vi "TractionModule Selection.vi"(8 "error in (no error)":errorcluster, 11 "Data Cluster":T1) -> (0 "error out":errorcluster)   [LabVIEW 2025]
uses:
  controls/LAB-IQ UI Data.ctl
  Traction Loop/Traction Receipe Enum.ctl
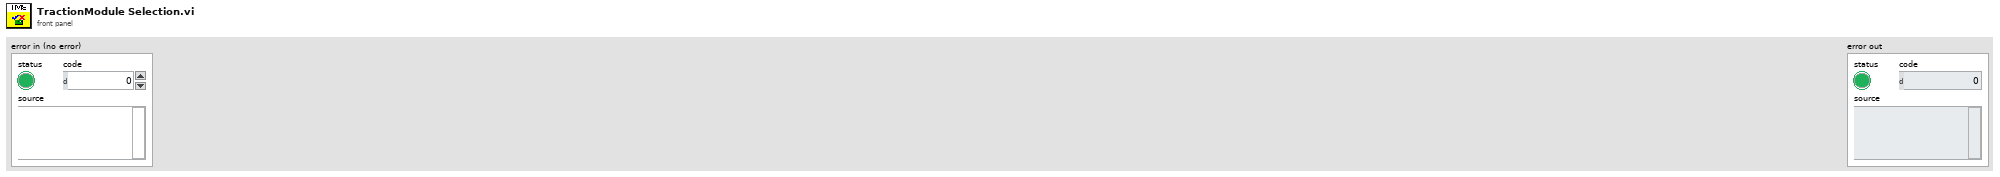
[diagram p1: front panel]
types:
  T1 = typedef "LAB-IQ UI Data.ctl" = cluster{"Main Home Screen":cluster{"GUI":refnum<vi>, "Platform Settings":refnum<vi>, "Configure":refnum<vi>, "Home":refnum<vi>, "EXIT":refnum<vi>, "service 2":refnum<vi>, "MainPage":refnum<vi>, "Analysis":refnum<vi>}, "Platform Settings":cluster{"mm/s  Surge":refnum<vi>, "Update Surge Speed":refnum<vi>, "Drive Error":refnum<vi>, "Disable Axis Jog Soft Limits":refnum<vi>, "mm/s  Sway":refnum<vi>, "Sway and Surge COM Status":refnum<vi>, "Heave COM Status":refnum<vi>, "Enable Platform":refnum<vi>, "Surge Forward Main":refnum<vi>, "Sway Right Main":refnum<vi>, "Sway Left Main":refnum<vi>, "Heave Down Main":refnum<vi>, "Heave Up main":refnum<vi>, "Update Sway Speed":refnum<vi>, "Update Heave Speed":refnum<vi>, "mm/s Heave":refnum<vi>, "mm/sec":refnum<vi>, "mm":refnum<vi>, "Surge Backward Main":refnum<vi>}, "Analysis Screen":cluster{"Analysis Home":refnum<vi>, "Surface Analysis":refnum<vi>, "Imaging":refnum<vi>, "Image Analysis":refnum<vi>, "Post Analysis":refnum<vi>}, "Config Screen":cluster{"Select Load Head":refnum<vi>, "Notes :":refnum<vi>, "FILE":refnum<vi>, "Sample ID :":refnum<vi>, "Operator ID :":refnum<vi>, "Operator Name :":refnum<vi>, "Auto":refnum<vi>}, "Motion Module":cluster{"zNL":refnum<vi>, "NL disp":refnum<vi>, "Rotary Tab":refnum<vi>, "Motion Direction:  3":refnum<vi>, "E.Velocity 2":refnum<vi>, "e.v/ssr 2":refnum<vi>, "Enter Fixed E.Velocity 2":refnum<vi>, "Enter Final SRR 2":refnum<vi>, "Enter initial SRR 2":refnum<vi>, "Enter Fixed SRR 2":refnum<vi>, "Enter the Final E.Velocity (m/s) 2":refnum<vi>, "Enter initial E.Velocity (m/s) 2":refnum<vi>, "Final Speed (RPM) 3":refnum<vi>, "Initial Speed (RPM) 2":refnum<vi>, "Enter the Final Velocity (m/s) 3":refnum<vi>, "Enter initial Velocity (m/s)  3":refnum<vi>, "Ramp Up 2":refnum<vi>, "TEST SELECTION":refnum<vi>, "SPEED SELECTION : ":refnum<vi>, "Angular Oscillation Set":refnum<vi>, "Traction":refnum<vi>, "Step Speed":refnum<vi>, "StepTable For Load-Speed":refnum<vi>, "StepTable For Speed":refnum<vi>, "Surge Forward MM":refnum<vi>, "Surge Backward MM":refnum<vi>, "M3 Image":refnum<vi>, "String 39":refnum<vi>, "Sway Left MM":refnum<vi>, "Sway Right MM":refnum<vi>, "Disable Axis Jog Soft Limits":refnum<vi>, "mm":refnum<vi>, "Heave Down MM":refnum<vi>, "Heave Up MM":refnum<vi>, "Wear Track Diameter (mm)":refnum<vi>, "Set WTD":refnum<vi>, "HomeScratch":refnum<vi>, "HomeRot":refnum<vi>, "PlaceModule":refnum<vi>, "Enter the Angle (Deg)":refnum<vi>, "Enter the Frequency (Hz)":refnum<vi>, "Motion Mode:":refnum<vi>, "LR Sway":refnum<vi>, "Rot Hor":refnum<vi>, "Scratch":refnum<vi>, "LR Cam":refnum<vi>, "MMBack":refnum<vi>, "MMNext":refnum<vi>, "Rot Ver":refnum<vi>, "Rotary Module Selection":refnum<vi>, "calculate rotary":refnum<vi>, "SPEED SELECTION : rotary":refnum<vi>, "Import 2":refnum<vi>, "Save 2":refnum<vi>, "File Path :  2":refnum<vi>, "String 45":refnum<vi>, "StepTable For Speed 3":refnum<vi>, "Enter the Speed(mm/sec)":refnum<vi>, "Enter the Speed(RPM)":refnum<vi>, "Enter Scratch Speed (mm/s):":refnum<vi>, "SwaySpeed Set":refnum<vi>, "Scartch Offset":refnum<vi>, "Motion type:":refnum<vi>, "HomeScratch 2":refnum<vi>, "Enter Scratch length (mm):":refnum<vi>, "Wear Track Diameter":refnum<vi>, "Rotary Speed Exced":refnum<vi>, "Scratch Mode":refnum<vi>, "No of Scratch":refnum<vi>}, "Environmental control":cluster{"Humidity  Status  3":refnum<vi>, "Low Temp  Status  2":refnum<vi>, "TK4 status 2":refnum<vi>, "Stage Temperature":refnum<vi>, "Sample Temperature":refnum<vi>, "Humidity (Amb)":refnum<vi>, "Clear List":refnum<vi>, "Add to list":refnum<vi>, "Wear":refnum<vi>, "Vibration":refnum<vi>, "Humidity (Chamber)":refnum<vi>, "Temperature (Chamber)":refnum<vi>, "ECR ":refnum<vi>, "Temperature (Amb)":refnum<vi>, "Microphone":refnum<vi>, "Acoustic Emission 3":refnum<vi>, "SNext":refnum<vi>, "APBack":refnum<vi>, "Enter the Temperature (°C):":refnum<vi>, "Enter the Stage \nTemperature (°C):":refnum<vi>, "Enter the Humidity (%Rh):":refnum<vi>, "Low Temp":refnum<vi>, "High Temp":refnum<vi>, "Humidity":refnum<vi>, "Sensors Picked":refnum<vi>}, "About Screen":cluster{"Password":refnum<vi>, "Home Service":refnum<vi>, "Advanced Setting":refnum<vi>, "About Tab":refnum<vi>, "ECR Port:":refnum<vi>, "Ramp Port:":refnum<vi>, "Installation/Replacement completed":refnum<vi>, "Loahead":refnum<vi>, "Heave and Surge COM Port:":refnum<vi>, "Sway COM Port:":refnum<vi>, "Temp Modbus:":refnum<vi>, "Humidity Port:":refnum<vi>, "Edit Gain Constants":refnum<vi>, "Save Gain Constants":refnum<vi>}, "Main Screen":cluster{"Main Screen Tab":refnum<vi>, "Angle and Frequency":refnum<vi>, "Stroke (mm)":refnum<vi>, "Angle (Deg)":refnum<vi>, "Main Speed Tab":refnum<vi>, "MTM MOTOR DISPLAY":refnum<vi>, "Disc Speed (m/sec)":refnum<vi>, "Ball Speed (m/sec)":refnum<vi>, "Disc Speed (RPM)":refnum<vi>, "Ball Speed (RPM)":refnum<vi>, "SPEED TAB":refnum<vi>, "Speed (m/sec)":refnum<vi>, "Set Speed (m/sec)":refnum<vi>, "Speed (RPM)":refnum<vi>, "Set Speed":refnum<vi>, "Time Tab":refnum<vi>, "Time ( HH:MM:SS ) 2":refnum<vi>, "Test Duration":refnum<vi>, "Test Duration 4":refnum<vi>, "TEST CYCLE":refnum<vi>, "TOTAL CYCLES":refnum<vi>, "Set Load (N)":refnum<vi>, "Temp Tabs":refnum<vi>, "Heater":refnum<vi>, "TK4 status":refnum<vi>, "ChamberTemp":refnum<vi>, "SetTmp":refnum<vi>, "Controller  Status":refnum<vi>, "ChamberTemp 2":refnum<vi>, "SetTmp 2":refnum<vi>, "Controller  Status 2":refnum<vi>, "ChamberTemp 3":refnum<vi>, "SetTmp 3":refnum<vi>, "Cooling":refnum<vi>, "Load Communication":refnum<vi>, "Ambient \nTemperature":refnum<vi>, "HumCOMStatus":refnum<vi>, "Ambient\n Humidity":refnum<vi>, "Freq (Hz)":refnum<vi>, "Load En":refnum<vi>, "NLt":refnum<vi>, "zNL 2":refnum<vi>, "Humidity On":refnum<vi>, "humidity disp":refnum<vi>, "Set Humidity":refnum<vi>, "NL disp 2":refnum<vi>, "Humidity On 2":refnum<vi>, "humidity disp 2":refnum<vi>, "Set Humidity 2":refnum<vi>, "NL disp 3":refnum<vi>, "AppLoadSeq scratch":refnum<vi>, "Stop Scratch":refnum<vi>, "ClrLog":refnum<vi>, "Trip Log":refnum<vi>, "STOP":refnum<vi>, "Start Test":refnum<vi>, "Test status":refnum<vi>, "AR Led":refnum<vi>, "Data":refnum<vi>, "Health":refnum<vi>, "Sway COM Status":refnum<vi>, "Heave COM Status":refnum<vi>, "Grp Tab":refnum<vi>, "Sub Graph":refnum<vi>, "SD (mm)":refnum<vi>, "Siliding distance Reset Graph":refnum<vi>, "SDGp":refnum<vi>, "Humidity Reset Graph":refnum<vi>, "HumrGp":refnum<vi>, "Acoustic Emission (mV)":refnum<vi>, "Aqucostic Reset Graph":refnum<vi>, "gACQUOS":refnum<vi>, "ECR RESET":refnum<vi>, "ECR":refnum<vi>, "Temperature Reset":refnum<vi>, "Acoustic Emission (mV) 2":refnum<vi>, "Aqucostic Reset Graph 2":refnum<vi>, "gACQUOS 2":refnum<vi>, "ECR RESET 2":refnum<vi>, "ECR 2":refnum<vi>, "Temperature Reset 2":refnum<vi>, "Temperature (deg c)":refnum<vi>, "Speed Reset Graph":refnum<vi>, "Speed Tab":refnum<vi>, "MTM DISC  SPEED":refnum<vi>, "MTM BALL SPEED":refnum<vi>, "speed mm/sec":refnum<vi>, "Hymidity":refnum<vi>, "Humidity Disable trip":refnum<vi>, "CoF Trip  2":refnum<vi>, "Depth Trip":refnum<vi>, "Weart Deapth":refnum<vi>, "Depth Reset Graph":refnum<vi>, "Weart":refnum<vi>, "Depthz":refnum<vi>, "Depth (µm)":refnum<vi>, "WearGp":refnum<vi>, "NL Trip 2":refnum<vi>, "Load pid":refnum<vi>, "Load Disable Trip":refnum<vi>, "Load Reset Graph":refnum<vi>, "NL Display 4":refnum<vi>, "Main Chart 3":refnum<vi>, "BACK":refnum<vi>, "Depth Trip 2":refnum<vi>, "COF TRIP ":refnum<vi>, "Friction Force (N)":refnum<vi>, "FF Reset Graph":refnum<vi>, "FF Disable Trip":refnum<vi>, "FF TRIP":refnum<vi>, "COF Disable Trip":refnum<vi>, "COF Reset Graph":refnum<vi>, "Start Test Temp":refnum<vi>, "zFF":refnum<vi>, "Friction Force (N) Graph":refnum<vi>, "Coefficient of Friction":refnum<vi>, "Scratch Start Test":refnum<vi>, "FF Tab":refnum<vi>, "Cyclic Friction Force (N)":refnum<vi>, "CZ FF":refnum<vi>, "Cyclic Friction Force (N) Graph":refnum<vi>, "Cyclic Coefficient of Friction":refnum<vi>, "Cyclic FF TRIP":refnum<vi>, "Cyclic FF Disable Trip":refnum<vi>, "cyclic COF Disable Trip":refnum<vi>, "cyclic COF TRIP":refnum<vi>, "cyclic COF Reset Graph":refnum<vi>, "Cyclic FF Reset Graph":refnum<vi>, "Test Trip":refnum<vi>, "Multi Scratch Pass":refnum<vi>, "Scratch Start Recording":refnum<vi>}, "Loading":cluster{"Indentation":refnum<vi>, "Reference Sample":refnum<vi>, "Load Cell Communication Slide":refnum<vi>, "com 3":refnum<vi>, "com":refnum<vi>, "DecaForce COM Status":refnum<vi>, "Update":refnum<vi>, "Clear 3":refnum<vi>, "seq":refnum<vi>, "Stribeck table":refnum<vi>, "Stribeck Table  For loading":refnum<vi>, "Loading Mode":refnum<vi>, "Enter the Final Load (N)":refnum<vi>, "Enter the CoF Trip":refnum<vi>, "Enter the Friction Force Trip":refnum<vi>, "Enter the Normal load Trip":refnum<vi>, "Enter the Load  (N)":refnum<vi>, "KiloForce":refnum<vi>, "DecaForce ":refnum<vi>, "MicroForce":refnum<vi>, "LHBack":refnum<vi>, "LHNext":refnum<vi>, "Enter the Loading Rate (N/min)":refnum<vi>, "Message":refnum<vi>, "Warning 2":refnum<vi>, "SSP 0.75":refnum<vi>, "SSP 0.5":refnum<vi>, "SSP 0.3":refnum<vi>, "Warning":refnum<vi>, "gui GIF":refnum<vi>, "Communication is established":refnum<vi>, "AppLoad 4":refnum<vi>, "Multipoint":refnum<vi>, "Load Selection":refnum<vi>}, "PID":cluster{"Ramp MulFac":refnum<vi>, "pulses LoadDiffRamp(2..10)":refnum<vi>, "PulseControlRamp(diff<=3N)":refnum<vi>, "SetLoadDeadband(%) Load(0-10N)":refnum<vi>, "PID gains out delay (microForce)":refnum<vi>, "Ramp":refnum<vi>, "Gain 2":refnum<vi>, "pulses LoadDiff(2..10)":refnum<vi>, "pulses LoadDiff(11..50)":refnum<vi>, "PulseControl(diff<=3N)":refnum<vi>, "SetLoadDeadband(%)  2":refnum<vi>, "Dummy Run":refnum<vi>, "Vertical load (N)":refnum<vi>, "AutoTune":refnum<vi>, "Offset 3 ":refnum<vi>, "apply load":refnum<vi>, "Offset  3":refnum<vi>, "apply load 2":refnum<vi>, "Enter ByPass Load":refnum<vi>, "reinit 3":refnum<vi>, "output range delay":refnum<vi>, "PID gains out delay":refnum<vi>, "Bypass Load":refnum<vi>, "pulsesSent":refnum<vi>, "pulses ":refnum<vi>, "actpid":refnum<vi>, "gFF Rot":refnum<vi>, "pulses LoadDiff(21..1000)":refnum<vi>, "Delay":refnum<vi>, "deadband":refnum<vi>}, "Config Parameters":cluster{"Tab Control 3":refnum<vi>, "Tab Control 19":refnum<vi>, "SAMPLES":refnum<vi>, "Re-initilaize":refnum<vi>, "Filter ON/OFF":refnum<vi>, "TracHomeSurgeOffsetCounts 10MM":refnum<vi>, "TracHomeSwayOffsetCounts 10MM":refnum<vi>, "Acoustic Emission:":refnum<vi>, "Apply Filter (FF)":refnum<vi>, "Filter% 2":refnum<vi>, "Apply Filter (Load)":refnum<vi>, "Filter% ":refnum<vi>, "Sway distance (mm)":refnum<vi>, "Surge distance (mm)":refnum<vi>, "DataSavingLoopDelay(ms)":refnum<vi>, "SAVE 2":refnum<vi>, "Enter Distance":refnum<vi>, "Sway Counts:":refnum<vi>, "Distance (mm): 3":refnum<vi>, "Surge Counts:":refnum<vi>, "Distance (mm): 2":refnum<vi>, "Distance (mm):":refnum<vi>, "Heave Counts:":refnum<vi>, "LRMHomeSurgeOffsetCounts":refnum<vi>, "LRMHomeSwayOffsetCounts":refnum<vi>, "TracHomeSurgeOffsetCounts 20MM":refnum<vi>, "TracHomeSwayOffsetCounts 20MM":refnum<vi>, "RotHomeSwayOffsetCounts":refnum<vi>, "RotHomeSurgeOffsetCounts":refnum<vi>, "Heave distance":refnum<vi>, "Zmm":refnum<vi>, "Heave Pulses/mm":refnum<vi>, "Surge Pulses/mm":refnum<vi>, "Sway Pulses/mm":refnum<vi>, "Heave Pitch":refnum<vi>, "Surge Pitch":refnum<vi>, "Sway Pitch":refnum<vi>, "Heave PPR":refnum<vi>, "Surge PPR":refnum<vi>, "Sway PPR":refnum<vi>, "Tab Control 5":refnum<vi>, "Tab Control 14":refnum<vi>, "Tab Control 26":refnum<vi>, "AE":refnum<vi>, "Heave Loop Delay":refnum<vi>, "Heave PID Speed":refnum<vi>, "Surge Jog Speed":refnum<vi>, "Heave Jog Speed":refnum<vi>, "Sway Loop Delay":refnum<vi>, "Sway PID Speed":refnum<vi>, "Sway Jog Speed":refnum<vi>, "DEPTH TRIP VALUE":refnum<vi>, "LOAD TRIP VALUE":refnum<vi>, "DEPTH TRIP   ENABLE":refnum<vi>, "LOAD TRIP  ENABLE":refnum<vi>, "CYCLIC FF TRIP VALUE":refnum<vi>, "FF TRIP VALUE":refnum<vi>, "CYCLIC CoF TRIP VALUE":refnum<vi>, "COF TRIP VALUE":refnum<vi>, "CYCLIC COF TRIP  ENABLE":refnum<vi>, "CYCLIC FF TRIP  ENABLE":refnum<vi>, "FF TRIP  ENABLE":refnum<vi>, "COF TRIP  ENABLE":refnum<vi>, "JOG TRIP LOAD VALUE (N)":refnum<vi>, "Rotary Vertical":refnum<vi>, "Traction":refnum<vi>, "Scratch":refnum<vi>, "LRM CAM":refnum<vi>, "Sway LRM":refnum<vi>, "Rotary Horizontal":refnum<vi>}, "Loading Com Port":cluster{"ClearAll":refnum<vi>, "Mz(Nm)":refnum<vi>, "My(Nm)":refnum<vi>, "Mx(Nm)":refnum<vi>, "Save Dwell":refnum<vi>, "Acq Delay (ms)":refnum<vi>, "Burst Delay (ms)":refnum<vi>, "model":refnum<vi>, "SN":refnum<vi>, "FFx(N)":refnum<vi>, "Sensor IP":refnum<vi>, "Port":refnum<vi>, "FFy(N)":refnum<vi>, "Load(N)":refnum<vi>, "delete Handle":refnum<vi>, "Create Handle":refnum<vi>, "ft_data":refnum<vi>, "ft_range":refnum<vi>, "ft_data 2":refnum<vi>, "stop 6":refnum<vi>, "running_flag":refnum<vi>, "ft_udp_handle":refnum<vi>, "get-data-return":refnum<vi>, "get-range-return":refnum<vi>, "zero-return":refnum<vi>, "filter-return":refnum<vi>, "initial-return":refnum<vi>, "deleteHandle-result":refnum<vi>, "Load Cell Temp":refnum<vi>, "Load Cell":refnum<vi>, "ZeroAll":refnum<vi>, "FORCE (N)":refnum<vi>, "TORQUE (N-m)":refnum<vi>}, "Heave AND Surge":cluster{"SURGE POSE":refnum<vi>, "error out Read":refnum<vi>, "HEAVE POSE":refnum<vi>, "State":refnum<vi>, "Homed":refnum<vi>, "Sequence ID":refnum<vi>, "error out Write":refnum<vi>, "faultCode":refnum<vi>, "Ack ID":refnum<vi>, "SPEED":refnum<vi>, "Distance":refnum<vi>, "Mode Command":refnum<vi>, "Heave and Surge Read":refnum<vi>, "Read Heave Temp":refnum<vi>, "Spare 15":refnum<vi>, "Spare 14":refnum<vi>, "Spare 13":refnum<vi>, "Spare 12":refnum<vi>, "Spare 11":refnum<vi>, "Spare 10":refnum<vi>, "Spare 9":refnum<vi>, "Spare 8":refnum<vi>, "Spare 7":refnum<vi>, "Spare 6":refnum<vi>, "Spare 5":refnum<vi>, "Spare 4":refnum<vi>, "Spare 2":refnum<vi>, "Spare 1":refnum<vi>, "Node Id":refnum<vi>, "Spare 3":refnum<vi>, "SPARE 4":refnum<vi>, "SPARE 3":refnum<vi>, "SPARE 2":refnum<vi>, "SPARE 1":refnum<vi>, "fwMajor":refnum<vi>, "fwMinor":refnum<vi>, "Manual Write":refnum<vi>, "Heave and Surge Write":refnum<vi>, "SPARE 5":refnum<vi>, "Reserved ":refnum<vi>, "SPARE 8":refnum<vi>, "SPARE 6":refnum<vi>, "SPARE 7":refnum<vi>, "SPARE 17":refnum<vi>, "SPARE 16":refnum<vi>, "SPARE 15":refnum<vi>, "SPARE 14":refnum<vi>, "SPARE 13":refnum<vi>, "SPARE 12":refnum<vi>, "SPARE 11":refnum<vi>, "SPARE 10":refnum<vi>, "SPARE 9":refnum<vi>, "System UPTIME":refnum<vi>, "Missed Packets":refnum<vi>, "faultCode Surge Right":refnum<vi>, "faultCode Surge Left":refnum<vi>, "faultCode Heave":refnum<vi>, "UPLINK HEAVE":refnum<vi>, "DOWNLINK HEAVE":refnum<vi>}, "New PID LOGIC":cluster{"Fine Tune Zone":refnum<vi>, "PID SDelay":refnum<vi>, "Max_pos_limit":refnum<vi>, "Min_pos_limit":refnum<vi>, "i_limit":refnum<vi>, "pct_scale":refnum<vi>, "Deadband":refnum<vi>, "Kd":refnum<vi>, "Ki":refnum<vi>, "Kp":refnum<vi>, "Current Position":refnum<vi>, "Set Load":refnum<vi>, "Current Load":refnum<vi>, "Pulse delta":refnum<vi>, "Init Step":refnum<vi>, "Max Step Linit":refnum<vi>, "min_deadband_floor":refnum<vi>, "dynamic_spindle_noise_scalar":refnum<vi>, "min_finetune_floor":refnum<vi>, "filter_alpha":refnum<vi>, "PID":refnum<vi>}, "SWAY ":cluster{"fwMajor":refnum<vi>, "Homed":refnum<vi>, "Rotary POSE":refnum<vi>, "State":refnum<vi>, "SWAY POSE":refnum<vi>, "Ack ID":refnum<vi>, "faultCode":refnum<vi>, "Node Id":refnum<vi>, "fwMinor":refnum<vi>, "Spare 6":refnum<vi>, "Spare 5":refnum<vi>, "Spare 4":refnum<vi>, "Spare 3":refnum<vi>, "Spare 2":refnum<vi>, "Spare 1":refnum<vi>, "Spare 7":refnum<vi>, "SPARE  5":refnum<vi>, "error out Write  SWAY ":refnum<vi>, "error out Read SWAY ":refnum<vi>, "Manual Write SWAY ":refnum<vi>, "SWAY WRITE":refnum<vi>, "SPARE  4":refnum<vi>, "SPARE  3":refnum<vi>, "SPARE 2":refnum<vi>, "SPARE 1":refnum<vi>, "Spare 15":refnum<vi>, "Spare 14":refnum<vi>, "Spare 13":refnum<vi>, "Spare 12":refnum<vi>, "Spare 11":refnum<vi>, "Spare 9":refnum<vi>, "Spare 8":refnum<vi>, "SPEED":refnum<vi>, "Distance":refnum<vi>, "Mode Command":refnum<vi>, "Sequence ID":refnum<vi>, "SWAY READ":refnum<vi>, "Spare 10":refnum<vi>, "Read SWAY Temp":refnum<vi>, "faultCode Sway ":refnum<vi>, "Missed Packets":refnum<vi>, "System UPTIME sway":refnum<vi>, "SPARE 6":refnum<vi>, "SPARE 7":refnum<vi>, "SPARE 9":refnum<vi>, "SPARE 11":refnum<vi>, "SPARE 10":refnum<vi>, "SPARE 8":refnum<vi>, "SPARE 13":refnum<vi>, "SPARE 12":refnum<vi>, "SPARE 17":refnum<vi>, "SPARE 16":refnum<vi>, "SPARE 15":refnum<vi>, "SPARE 14":refnum<vi>, "Reserved":refnum<vi>, "faultCode Rotary":refnum<vi>, "UPLINK SWAY":refnum<vi>, "DOWNLINK SWAY":refnum<vi>}, "Analysis Screen":cluster{"Analysis Home":refnum<vi>, "Refresh 2":refnum<vi>, "MEAN 4":refnum<vi>, "SD 4":refnum<vi>, "VARIANCE 4":refnum<vi>, "MEAN  3":refnum<vi>, "SD  3":refnum<vi>, "VARIANCE  3":refnum<vi>, "MEAN 2":refnum<vi>, "SD  2":refnum<vi>, "VARIANCE 2":refnum<vi>, "MEAN":refnum<vi>, "SD":refnum<vi>, "VARIANCE":refnum<vi>, "File 4 Discription":refnum<vi>, "OPEN 4":refnum<vi>, "File Name 4":refnum<vi>, "OPEN 3":refnum<vi>, "File 3 Discription":refnum<vi>, "File Name 3":refnum<vi>, "Y-AXIS":refnum<vi>, "X-AXIS":refnum<vi>, "XY Graph":refnum<vi>, "File Name 2":refnum<vi>, "File Name 1":refnum<vi>, "OPEN 2":refnum<vi>, "OPEN 1":refnum<vi>, "File 1 Discription ":refnum<vi>, "File 2 Discription":refnum<vi>, "Export":refnum<vi>, "File Format":refnum<vi>}, "Traction":cluster{"faultCode Traction 2":refnum<vi>, "faultCode Traction 1":refnum<vi>, "Missed Packets":refnum<vi>, "System UPTIME Traction":refnum<vi>, "SPARE 17":refnum<vi>, "SPARE 16":refnum<vi>, "SPARE 15":refnum<vi>, "SPARE 14":refnum<vi>, "SPARE 13":refnum<vi>, "SPARE 12":refnum<vi>, "SPARE 11":refnum<vi>, "SPARE 10":refnum<vi>, "SPARE 9":refnum<vi>, "SPARE 8":refnum<vi>, "SPARE 7":refnum<vi>, "SPARE 6":refnum<vi>, "Reserved":refnum<vi>, "SPARE  5":refnum<vi>, "Manual Write TRACTION":refnum<vi>, "TRACTION WRITE":refnum<vi>, "SPARE  4":refnum<vi>, "SPARE  3":refnum<vi>, "SPARE 2":refnum<vi>, "SPARE 1":refnum<vi>, "Spare 7":refnum<vi>, "Spare 6":refnum<vi>, "Spare 5":refnum<vi>, "Spare 4":refnum<vi>, "Spare 2":refnum<vi>, "Spare 1":refnum<vi>, "Node Id":refnum<vi>, "Read TRACTION Temp":refnum<vi>, "fwMinor":refnum<vi>, "fwMajor":refnum<vi>, "faultCode":refnum<vi>, "TRACTION POSE":refnum<vi>, "TRACTION POSE 2":refnum<vi>, "Homed":refnum<vi>, "State":refnum<vi>, "Ack ID":refnum<vi>, "SPEED":refnum<vi>, "Distance":refnum<vi>, "Mode Command":refnum<vi>, "Sequence ID":refnum<vi>, "error out Read TRACTION":refnum<vi>, "error out Write  TRACTION":refnum<vi>, "TRACTION READ":refnum<vi>, "Spare 3":refnum<vi>, "Downlink traction":refnum<vi>, "Uplink Traction":refnum<vi>}, "Traction reciepe":cluster{"SRR Sweep Range (%) Stribeck":refnum<vi>, "Traction Receipe":refnum<vi>, "Total Execution Time":refnum<vi>, "Total Steps":refnum<vi>, "Duration / Step (s)  Stribeck":refnum<vi>, "STRIBECK Fixed SRR List (%)":refnum<vi>, "Duration / Step (s) Traction":refnum<vi>, "SRR Sweep Range (%) traction":refnum<vi>, "Rolling Speed (mm/s)":refnum<vi>, "Temperature Stages (°C)":refnum<vi>, "Ball Load (N)":refnum<vi>, "Lubricant Name":refnum<vi>, "Profile File Name":refnum<vi>, "SET entrainment Velocity":refnum<vi>, "Test Array Size":refnum<vi>, "SRR INDEX [ STRIBECK]":refnum<vi>, "Stribeck Size":refnum<vi>, "SET SRR":refnum<vi>, "ELAPSED TIMER ":refnum<vi>, "BALL SET RPM":refnum<vi>, "DISC SET RPM":refnum<vi>, "SET LOAD":refnum<vi>, "TEMPERATURE READ":refnum<vi>, "SET TEMPERATURE":refnum<vi>, "Traction Size":refnum<vi>, "DISC SPEED (rpm)":refnum<vi>, "BALL SPEED (rpm)":refnum<vi>, "BALL WEAR TRACK":refnum<vi>, "DISC WEARTRACK":refnum<vi>, "SRR INDEX [ TRACTION]":refnum<vi>, "Start Index Type":refnum<vi>, "Enum - Menu":refnum<vi>, "Ball (mm/sec)":refnum<vi>, "Disc (mm/sec)":refnum<vi>}, "Traction Control":cluster{"HomeTraction":refnum<vi>, "Demo Mode Display":refnum<vi>, "Traction Message":refnum<vi>, "Traction Step Update Details":refnum<vi>, "Main Tab sequence for selection":refnum<vi>, "Ramp Tab":refnum<vi>, "e.v/ssr":refnum<vi>, "Enter Fixed E.Velocity":refnum<vi>, "Enter Final SRR":refnum<vi>, "Enter initial SRR":refnum<vi>, "Enter Fixed SRR":refnum<vi>, "Enter the Final E.Velocity (m/s)":refnum<vi>, "Enter initial E.Velocity (m/s)":refnum<vi>, "Ball WTD":refnum<vi>, "E.Velocity":refnum<vi>, "Enter the Final Velocity (m/s)":refnum<vi>, "Enter initial Velocity (m/s)":refnum<vi>, "Ramp Up   Disc":refnum<vi>, "Initial DiscSpeed (RPM)":refnum<vi>, "Final Speed (RPM) Ball":refnum<vi>, "Final Speed (RPM)":refnum<vi>, "Initial Speed (RPM) Ball":refnum<vi>, "Enter the Final Velocity (m/s) Ball":refnum<vi>, "Enter initial Velocity (m/s) Ball":refnum<vi>, "Ramp Up":refnum<vi>, "ExceedBallSpeed step":refnum<vi>, "ExceedDiscSpeed":refnum<vi>, "BallSpeed Exceed Indication":refnum<vi>, "Apply":refnum<vi>, "SPEED SELECTION : MTM":refnum<vi>, "SPEED SELECTION : MTM 2":refnum<vi>, "TEST SELECTION (MTM)":refnum<vi>, "MTM Test Selection":refnum<vi>, "File Path Tab":refnum<vi>, "File Path String":refnum<vi>, "Save":refnum<vi>, "Save  2":refnum<vi>, "Import ":refnum<vi>, "File Path :":refnum<vi>, "Step Sequence Indication Tab":refnum<vi>, "Step Sequence Indication":refnum<vi>, "Calculate Step":refnum<vi>, "StepTable":refnum<vi>, "ExceedDiscSpeed  Cinstant Speed":refnum<vi>, "ExceedBallSpeed Constant":refnum<vi>, "TEST SELECTION (MTM) 2":refnum<vi>, "SPEED SELECTION : MTM 3":refnum<vi>, "MTM Test Selection 2":refnum<vi>, "Enter the Speed (m/sec): ":refnum<vi>, "Enter the Speed (m/sec):  2":refnum<vi>, "Enter the Speed (RPM):":refnum<vi>, "Lower Spped ":refnum<vi>, "Upper":refnum<vi>, "Enter the Speed (RPM):Ball":refnum<vi>, "Disc Motion Direction: ":refnum<vi>, "Ball Motion Direction :":refnum<vi>, "Motion Mode: ":refnum<vi>, "Wear Track Diameter (mm) ":refnum<vi>, "Disc Speed Indicator":refnum<vi>, "ExceedBallSpeed":refnum<vi>}, "Acquostic":cluster{"Last Config Rejected ":refnum<vi>, "rx command count":refnum<vi>, "Current Filter Id":refnum<vi>, "Isolated Gain":refnum<vi>, "DAQ Status":refnum<vi>, "error out":refnum<vi>, "error in (no error)":refnum<vi>, "Uplink Packet":refnum<vi>, "data out":refnum<vi>, "Downlink Packet":refnum<vi>, "Signal Energy":refnum<vi>, "Amplitude db_AE":refnum<vi>, "Peak Amplitude":refnum<vi>, "AE Ring-Down Counts":refnum<vi>, "Gains":refnum<vi>, "Manual Write Acquostic":refnum<vi>}}
  T2 = enum32{"Details", "PlatformSetting", "Analysis", "HOME"}
  T3 = enum32{"Setup", "Load Head", "Motion Module", "Environment", "Begin"}
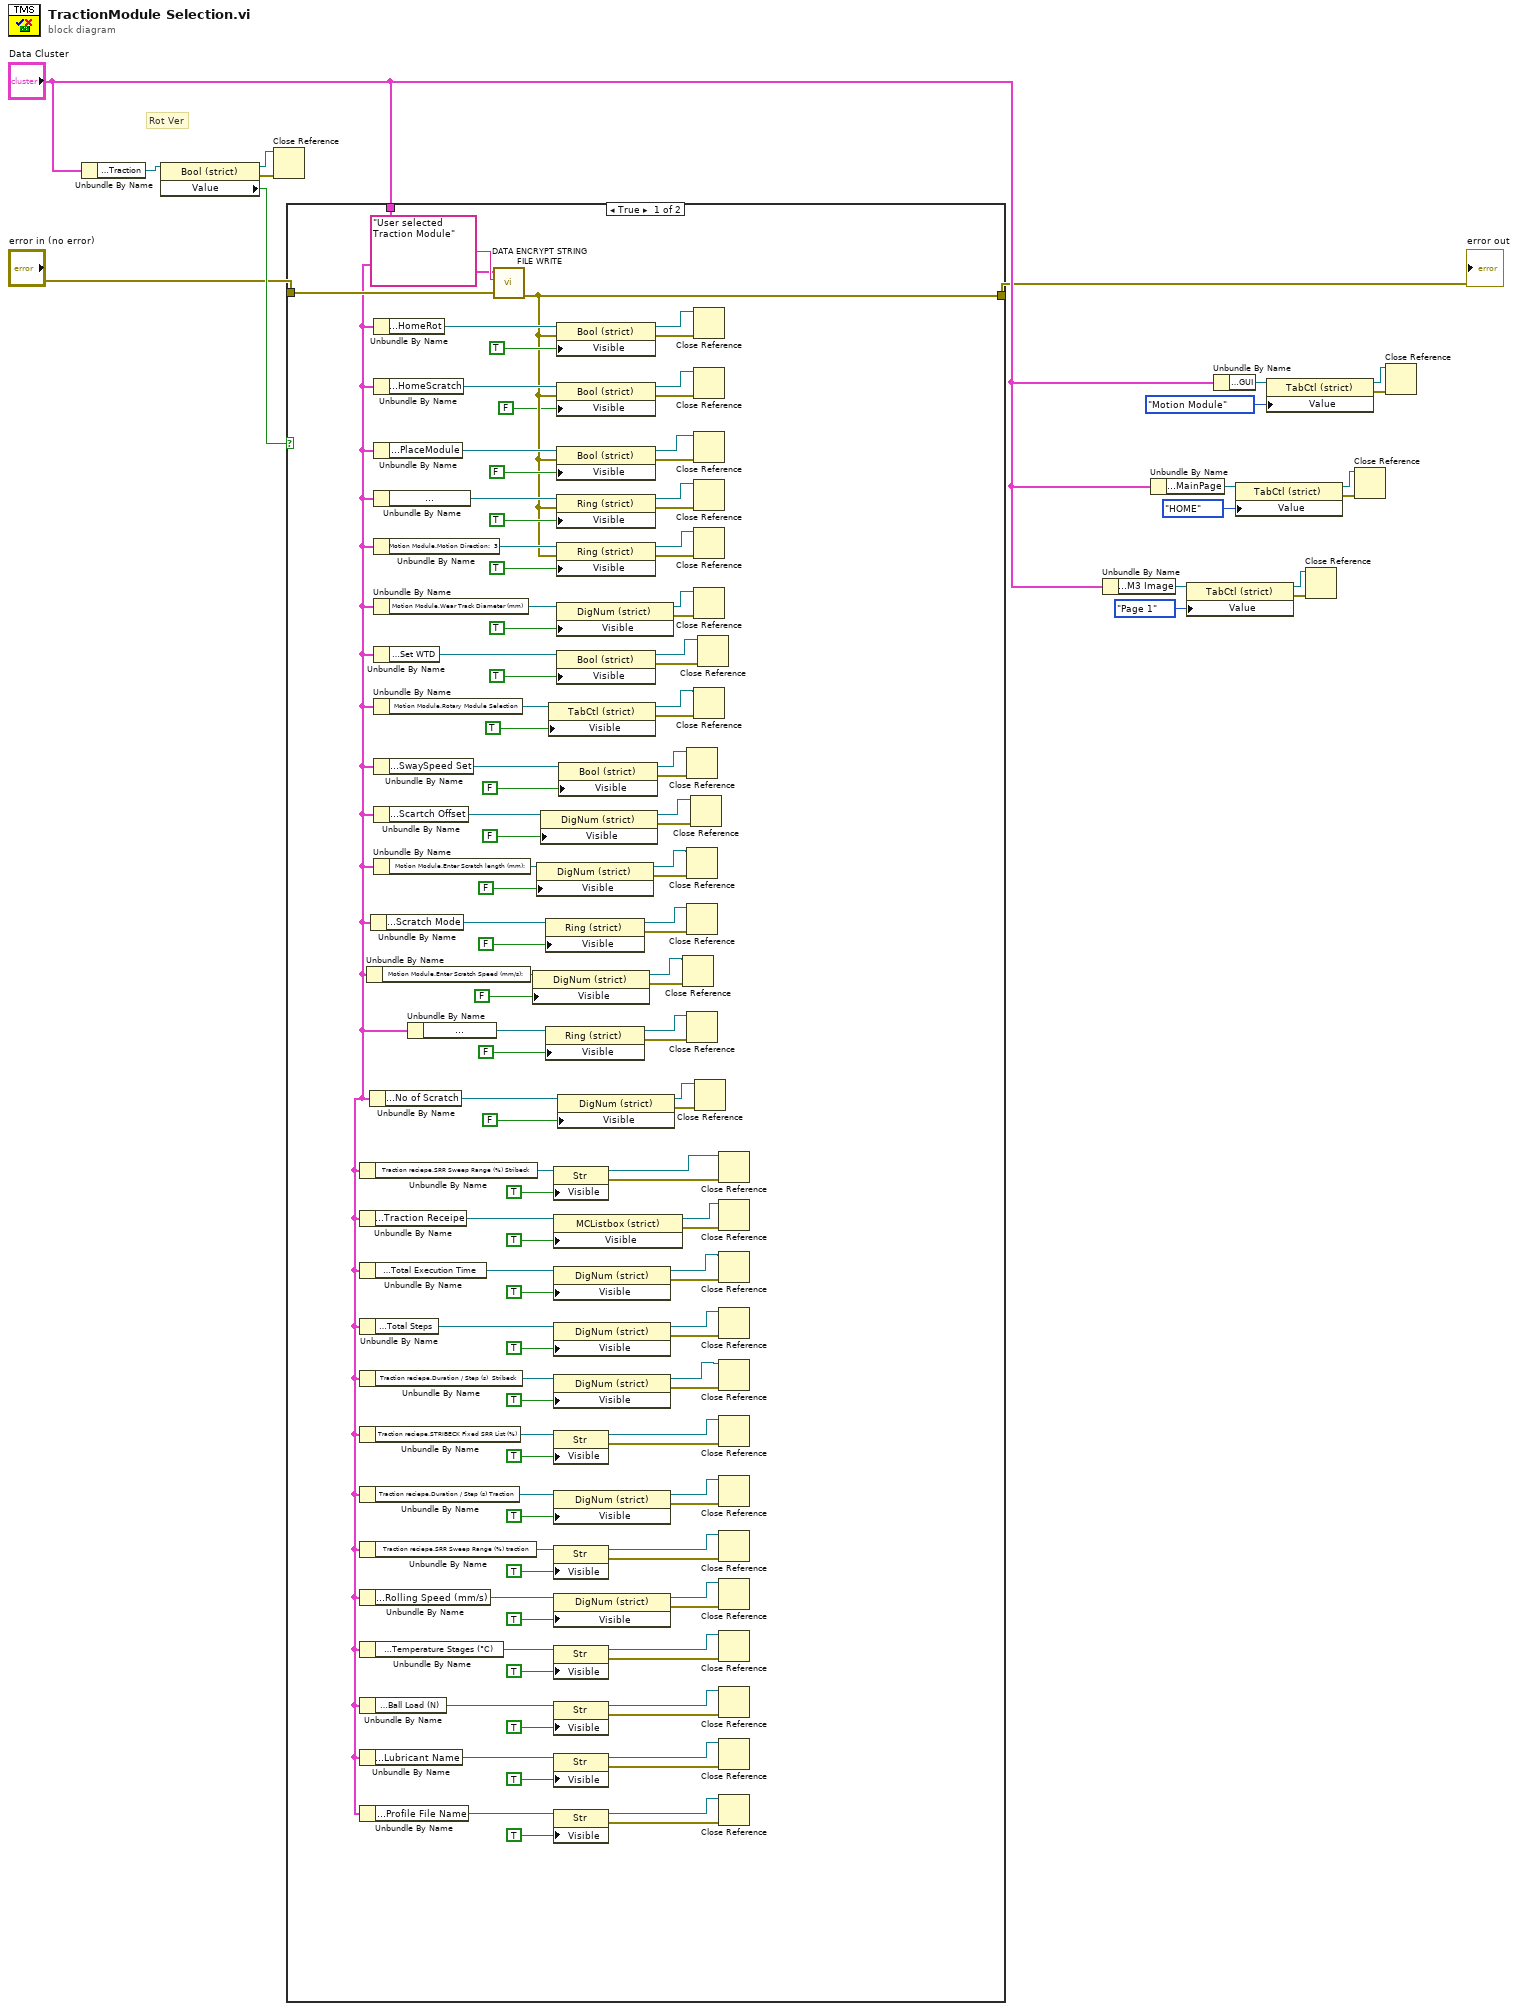
[diagram p0: block diagram]
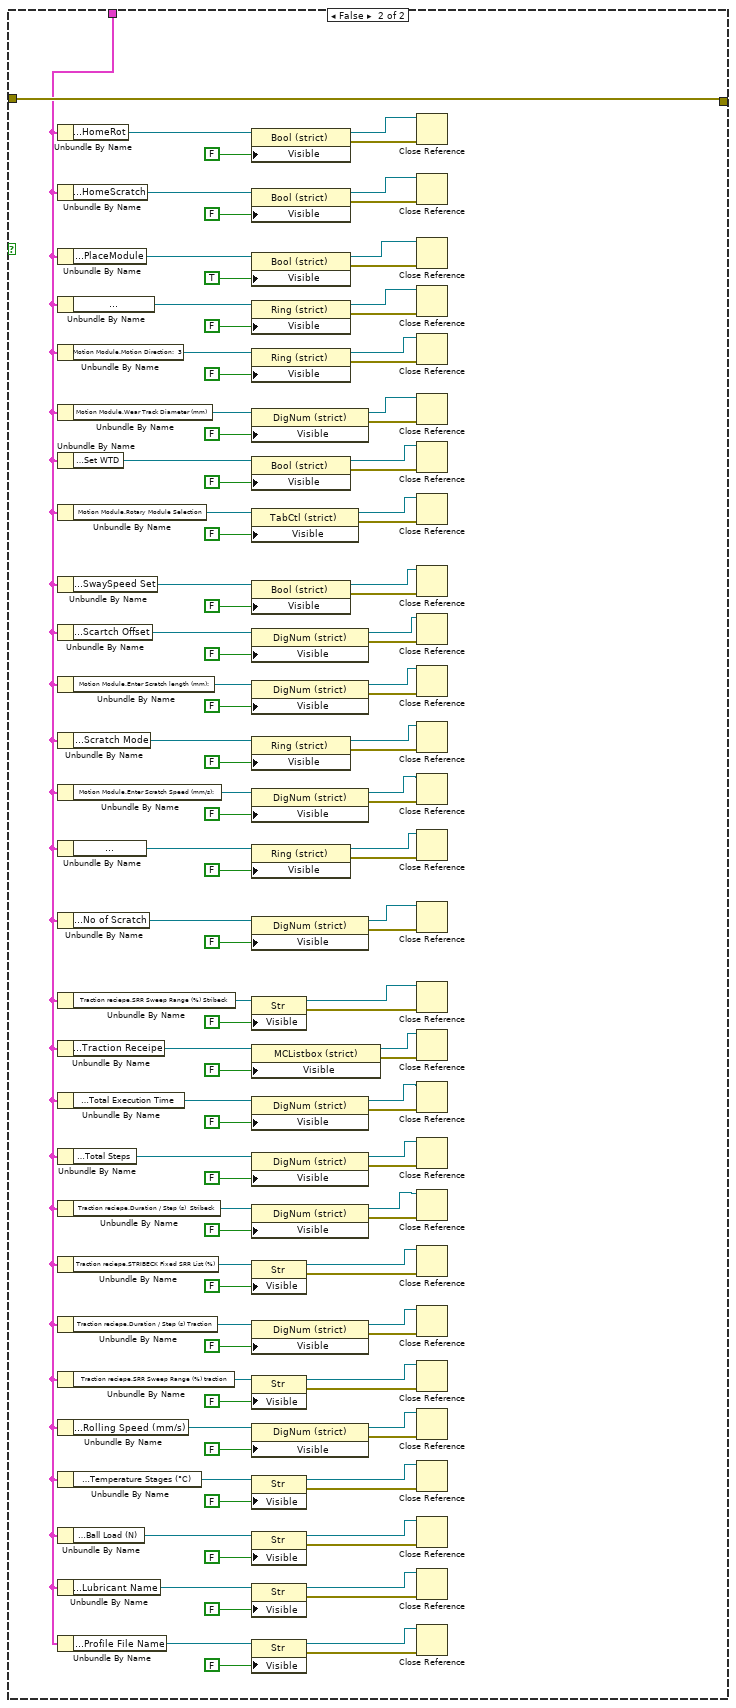
[diagram p2: hidden frame]
diagram:
  # "Rot Ver"
  n1 = Unbundle By Name("Data Cluster") -> ("Motion Module.Traction"=w18:refnum<vi>)
  n2 = property class="Bool (strict)"(reference=w18) -> (reference out=w15:refnum<vi>, error out=w16:errorcluster, "Value"=w19:bool)  [unwired: 1 in]
  n3 = Close Reference(reference=w15, error in (no error)=w16) -> ()  [unwired: 1 out]
  n4 = case shown="True" w19 {
    tunnel: "error in (no error)" -> [w134 w249]
    tunnel: [w106 w249] -> w10
    tunnel: "Data Cluster" -> [w20 w136]
    frame True {
      n5 = Unbundle By Name(w20) -> ("Traction reciepe.SRR Sweep Range (%) Stribeck"=w55:refnum<vi>)
      n6 = Unbundle By Name(w20) -> ("Traction reciepe.Traction Receipe"=w58:refnum<vi>)
      n7 = Unbundle By Name(w20) -> ("Traction reciepe.Total Execution Time"=w61:refnum<vi>)
      n8 = Unbundle By Name(w20) -> ("Traction reciepe.Total Steps"=w53:refnum<vi>)
      n9 = Unbundle By Name(w20) -> ("Traction reciepe.Duration / Step (s)  Stribeck"=w50:refnum<vi>)
      n10 = Unbundle By Name(w20) -> ("Traction reciepe.STRIBECK Fixed SRR List (%)"=w47:refnum<vi>)
      n11 = Unbundle By Name(w20) -> ("Traction reciepe.Duration / Step (s) Traction"=w70:refnum<vi>)
      n12 = Unbundle By Name(w20) -> ("Traction reciepe.SRR Sweep Range (%) traction"=w34:refnum<vi>)
      n13 = Unbundle By Name(w20) -> ("Traction reciepe.Rolling Speed (mm/s)"=w31:refnum<vi>)
      n14 = Unbundle By Name(w20) -> ("Traction reciepe.Temperature Stages (°C)"=w28:refnum<vi>)
      n15 = Unbundle By Name(w20) -> ("Traction reciepe.Ball Load (N)"=w36:refnum<vi>)
      n16 = Unbundle By Name(w20) -> ("Traction reciepe.Lubricant Name"=w39:refnum<vi>)
      n17 = Unbundle By Name(w20) -> ("Traction reciepe.Profile File Name"=w42:refnum<vi>)
      n18 = Unbundle By Name(w20) -> ("Motion Module.Enter Scratch Speed (mm/s):"=w83:refnum<vi>)
      n19 = Unbundle By Name(w20) -> ("Motion Module.No of Scratch"=w75:refnum<vi>)
      n20 = Unbundle By Name(w20) -> ("Motion Module.Scratch Mode"=w88:refnum<vi>)
      n21 = Unbundle By Name(w20) -> ("Motion Module.HomeRot"=w133:refnum<vi>)
      n22 = Unbundle By Name(w20) -> ("Motion Module.HomeScratch"=w128:refnum<vi>)
      n23 = Unbundle By Name(w20) -> ("Motion Module.PlaceModule"=w126:refnum<vi>)
      n24 = Unbundle By Name(w20) -> ("Motion Module.Motion Mode:"=w119:refnum<vi>)
      n25 = Unbundle By Name(w20) -> ("Motion Module.Motion Direction:  3"=w118:refnum<vi>)
      n26 = Unbundle By Name(w20) -> ("Motion Module.Wear Track Diameter (mm)"=w112:refnum<vi>)
      n27 = Unbundle By Name(w20) -> ("Motion Module.Set WTD"=w109:refnum<vi>)
      n28 = Unbundle By Name(w20) -> ("Motion Module.Rotary Module Selection"=w103:refnum<vi>)
      n29 = Unbundle By Name(w20) -> ("Motion Module.SwaySpeed Set"=w91:refnum<vi>)
      n30 = Unbundle By Name(w20) -> ("Motion Module.Scartch Offset"=w94:refnum<vi>)
      n31 = Unbundle By Name(w20) -> ("Motion Module.Enter Scratch length (mm):"=w99:refnum<vi>)
      n32 = Unbundle By Name(w20) -> ("Motion Module.Motion type:"=w80:refnum<vi>)
      n33 = call "DATA ENCRYPT STRING FILE WRITE.vi"("error in (no error)"=w134, "User Action"="User selected Traction Module", "main ref"=w20) -> ("error out"=w106:errorcluster)  [unwired: 6 in, 1 out]
      n34 = property class="DigNum (strict)"(reference=w83, "Visible"=FALSE) -> (reference out=w82:refnum<vi>, error out=w84:errorcluster)  [unwired: 1 in]
      n35 = property class="DigNum (strict)"(reference=w99, "Visible"=FALSE) -> (reference out=w100:refnum<vi>, error out=w98:errorcluster)  [unwired: 1 in]
      n36 = property class="DigNum (strict)"(reference=w94, "Visible"=FALSE) -> (reference out=w93:refnum<vi>, error out=w95:errorcluster)  [unwired: 1 in]
      n37 = property class="Ring (strict)"(reference=w88, "Visible"=FALSE) -> (reference out=w81:refnum<vi>, error out=w87:errorcluster)  [unwired: 1 in]
      n38 = property class="Ring (strict)"(reference=w80, "Visible"=FALSE) -> (reference out=w77:refnum<vi>, error out=w79:errorcluster)  [unwired: 1 in]
      n39 = property class="TabCtl (strict)"(reference=w103, "Visible"=TRUE) -> (reference out=w102:refnum<vi>, error out=w104:errorcluster)  [unwired: 1 in]
      n40 = property class="Str"(reference=w55, "Visible"=TRUE) -> (reference out=w56:refnum<vi>, error out=w54:errorcluster)  [unwired: 1 in]
      n41 = property class="MCListbox (strict)"(reference=w58, "Visible"=TRUE) -> (reference out=w57:refnum<vi>, error out=w59:errorcluster)  [unwired: 1 in]
      n42 = property class="DigNum (strict)"(reference=w61, "Visible"=TRUE) -> (reference out=w62:refnum<vi>, error out=w60:errorcluster)  [unwired: 1 in]
      n43 = property class="DigNum (strict)"(reference=w53, "Visible"=TRUE) -> (reference out=w48:refnum<vi>, error out=w52:errorcluster)  [unwired: 1 in]
      n44 = property class="DigNum (strict)"(reference=w50, "Visible"=TRUE) -> (reference out=w49:refnum<vi>, error out=w51:errorcluster)  [unwired: 1 in]
      n45 = property class="Str"(reference=w47, "Visible"=TRUE) -> (reference out=w45:refnum<vi>, error out=w46:errorcluster)  [unwired: 1 in]
      n46 = property class="DigNum (strict)"(reference=w70, "Visible"=TRUE) -> (reference out=w72:refnum<vi>, error out=w71:errorcluster)  [unwired: 1 in]
      n47 = property class="Str"(reference=w34, "Visible"=TRUE) -> (reference out=w33:refnum<vi>, error out=w35:errorcluster)  [unwired: 1 in]
      n48 = property class="DigNum (strict)"(reference=w31, "Visible"=TRUE) -> (reference out=w32:refnum<vi>, error out=w30:errorcluster)  [unwired: 1 in]
      n49 = property class="Str"(reference=w28, "Visible"=TRUE) -> (reference out=w27:refnum<vi>, error out=w29:errorcluster)  [unwired: 1 in]
      n50 = property class="Str"(reference=w36, "Visible"=TRUE) -> (reference out=w41:refnum<vi>, error out=w37:errorcluster)  [unwired: 1 in]
      n51 = property class="Str"(reference=w39, "Visible"=TRUE) -> (reference out=w40:refnum<vi>, error out=w38:errorcluster)  [unwired: 1 in]
      n52 = property class="Str"(reference=w42, "Visible"=TRUE) -> (reference out=w44:refnum<vi>, error out=w43:errorcluster)  [unwired: 1 in]
      n53 = property class="Bool (strict)"(reference=w133, error in=w106, "Visible"=TRUE) -> (reference out=w131:refnum<vi>, error out=w132:errorcluster)
      n54 = property class="Bool (strict)"(reference=w128, error in=w106, "Visible"=FALSE) -> (reference out=w130:refnum<vi>, error out=w129:errorcluster)
      n55 = property class="Bool (strict)"(reference=w126, error in=w106, "Visible"=FALSE) -> (reference out=w124:refnum<vi>, error out=w125:errorcluster)
      n56 = property class="Ring (strict)"(reference=w119, error in=w106, "Visible"=TRUE) -> (reference out=w121:refnum<vi>, error out=w120:errorcluster)
      n57 = property class="Ring (strict)"(reference=w118, error in=w106, "Visible"=TRUE) -> (reference out=w115:refnum<vi>, error out=w117:errorcluster)
      n58 = property class="DigNum (strict)"(reference=w112, "Visible"=TRUE) -> (reference out=w111:refnum<vi>, error out=w113:errorcluster)  [unwired: 1 in]
      n59 = property class="Bool (strict)"(reference=w109, "Visible"=TRUE) -> (reference out=w110:refnum<vi>, error out=w108:errorcluster)  [unwired: 1 in]
      n60 = property class="DigNum (strict)"(reference=w75, "Visible"=FALSE) -> (reference out=w73:refnum<vi>, error out=w74:errorcluster)  [unwired: 1 in]
      n61 = property class="Bool (strict)"(reference=w91, "Visible"=FALSE) -> (reference out=w92:refnum<vi>, error out=w90:errorcluster)  [unwired: 1 in]
      n62 = Close Reference(reference=w82, error in (no error)=w84) -> ()  [unwired: 1 out]
      n63 = Close Reference(reference=w92, error in (no error)=w90) -> ()  [unwired: 1 out]
      n64 = Close Reference(reference=w100, error in (no error)=w98) -> ()  [unwired: 1 out]
      n65 = Close Reference(reference=w81, error in (no error)=w87) -> ()  [unwired: 1 out]
      n66 = Close Reference(reference=w77, error in (no error)=w79) -> ()  [unwired: 1 out]
      n67 = Close Reference(reference=w93, error in (no error)=w95) -> ()  [unwired: 1 out]
      n68 = Close Reference(reference=w131, error in (no error)=w132) -> ()  [unwired: 1 out]
      n69 = Close Reference(reference=w130, error in (no error)=w129) -> ()  [unwired: 1 out]
      n70 = Close Reference(reference=w124, error in (no error)=w125) -> ()  [unwired: 1 out]
      n71 = Close Reference(reference=w121, error in (no error)=w120) -> ()  [unwired: 1 out]
      n72 = Close Reference(reference=w115, error in (no error)=w117) -> ()  [unwired: 1 out]
      n73 = Close Reference(reference=w111, error in (no error)=w113) -> ()  [unwired: 1 out]
      n74 = Close Reference(reference=w102, error in (no error)=w104) -> ()  [unwired: 1 out]
      n75 = Close Reference(reference=w73, error in (no error)=w74) -> ()  [unwired: 1 out]
      n76 = Close Reference(reference=w110, error in (no error)=w108) -> ()  [unwired: 1 out]
      n77 = Close Reference(reference=w56, error in (no error)=w54) -> ()  [unwired: 1 out]
      n78 = Close Reference(reference=w57, error in (no error)=w59) -> ()  [unwired: 1 out]
      n79 = Close Reference(reference=w62, error in (no error)=w60) -> ()  [unwired: 1 out]
      n80 = Close Reference(reference=w48, error in (no error)=w52) -> ()  [unwired: 1 out]
      n81 = Close Reference(reference=w49, error in (no error)=w51) -> ()  [unwired: 1 out]
      n82 = Close Reference(reference=w45, error in (no error)=w46) -> ()  [unwired: 1 out]
      n83 = Close Reference(reference=w72, error in (no error)=w71) -> ()  [unwired: 1 out]
      n84 = Close Reference(reference=w33, error in (no error)=w35) -> ()  [unwired: 1 out]
      n85 = Close Reference(reference=w32, error in (no error)=w30) -> ()  [unwired: 1 out]
      n86 = Close Reference(reference=w27, error in (no error)=w29) -> ()  [unwired: 1 out]
      n87 = Close Reference(reference=w41, error in (no error)=w37) -> ()  [unwired: 1 out]
      n88 = Close Reference(reference=w40, error in (no error)=w38) -> ()  [unwired: 1 out]
      n89 = Close Reference(reference=w44, error in (no error)=w43) -> ()  [unwired: 1 out]
    }
    frame False {
      n90 = Unbundle By Name(w136) -> ("Motion Module.HomeRot"=w248:refnum<vi>)
      n91 = Unbundle By Name(w136) -> ("Motion Module.HomeScratch"=w243:refnum<vi>)
      n92 = Unbundle By Name(w136) -> ("Motion Module.PlaceModule"=w241:refnum<vi>)
      n93 = Unbundle By Name(w136) -> ("Motion Module.Motion Mode:"=w234:refnum<vi>)
      n94 = Unbundle By Name(w136) -> ("Motion Module.Motion Direction:  3"=w233:refnum<vi>)
      n95 = Unbundle By Name(w136) -> ("Motion Module.Wear Track Diameter (mm)"=w227:refnum<vi>)
      n96 = Unbundle By Name(w136) -> ("Motion Module.Set WTD"=w224:refnum<vi>)
      n97 = Unbundle By Name(w136) -> ("Motion Module.Rotary Module Selection"=w219:refnum<vi>)
      n98 = Unbundle By Name(w136) -> ("Motion Module.SwaySpeed Set"=w206:refnum<vi>)
      n99 = Unbundle By Name(w136) -> ("Motion Module.Scartch Offset"=w203:refnum<vi>)
      n100 = Unbundle By Name(w136) -> ("Motion Module.Enter Scratch length (mm):"=w200:refnum<vi>)
      n101 = Unbundle By Name(w136) -> ("Motion Module.Scratch Mode"=w208:refnum<vi>)
      n102 = Unbundle By Name(w136) -> ("Motion Module.Enter Scratch Speed (mm/s):"=w211:refnum<vi>)
      n103 = Unbundle By Name(w136) -> ("Motion Module.Motion type:"=w214:refnum<vi>)
      n104 = Unbundle By Name(w136) -> ("Motion Module.No of Scratch"=w191:refnum<vi>)
      n105 = Unbundle By Name(w136) -> ("Traction reciepe.SRR Sweep Range (%) Stribeck"=w171:refnum<vi>)
      n106 = Unbundle By Name(w136) -> ("Traction reciepe.Traction Receipe"=w174:refnum<vi>)
      n107 = Unbundle By Name(w136) -> ("Traction reciepe.Total Execution Time"=w177:refnum<vi>)
      n108 = Unbundle By Name(w136) -> ("Traction reciepe.Total Steps"=w169:refnum<vi>)
      n109 = Unbundle By Name(w136) -> ("Traction reciepe.Duration / Step (s)  Stribeck"=w166:refnum<vi>)
      n110 = Unbundle By Name(w136) -> ("Traction reciepe.STRIBECK Fixed SRR List (%)"=w163:refnum<vi>)
      n111 = Unbundle By Name(w136) -> ("Traction reciepe.Duration / Step (s) Traction"=w186:refnum<vi>)
      n112 = Unbundle By Name(w136) -> ("Traction reciepe.SRR Sweep Range (%) traction"=w150:refnum<vi>)
      n113 = Unbundle By Name(w136) -> ("Traction reciepe.Rolling Speed (mm/s)"=w147:refnum<vi>)
      n114 = Unbundle By Name(w136) -> ("Traction reciepe.Temperature Stages (°C)"=w144:refnum<vi>)
      n115 = Unbundle By Name(w136) -> ("Traction reciepe.Ball Load (N)"=w152:refnum<vi>)
      n116 = Unbundle By Name(w136) -> ("Traction reciepe.Lubricant Name"=w155:refnum<vi>)
      n117 = Unbundle By Name(w136) -> ("Traction reciepe.Profile File Name"=w158:refnum<vi>)
      n118 = property class="Bool (strict)"(reference=w248, "Visible"=FALSE) -> (reference out=w246:refnum<vi>, error out=w247:errorcluster)  [unwired: 1 in]
      n119 = property class="Bool (strict)"(reference=w243, "Visible"=FALSE) -> (reference out=w245:refnum<vi>, error out=w244:errorcluster)  [unwired: 1 in]
      n120 = property class="Bool (strict)"(reference=w241, "Visible"=TRUE) -> (reference out=w239:refnum<vi>, error out=w240:errorcluster)  [unwired: 1 in]
      n121 = property class="Ring (strict)"(reference=w234, "Visible"=FALSE) -> (reference out=w236:refnum<vi>, error out=w235:errorcluster)  [unwired: 1 in]
      n122 = property class="Ring (strict)"(reference=w233, "Visible"=FALSE) -> (reference out=w230:refnum<vi>, error out=w232:errorcluster)  [unwired: 1 in]
      n123 = property class="DigNum (strict)"(reference=w227, "Visible"=FALSE) -> (reference out=w226:refnum<vi>, error out=w228:errorcluster)  [unwired: 1 in]
      n124 = property class="Bool (strict)"(reference=w224, "Visible"=FALSE) -> (reference out=w225:refnum<vi>, error out=w223:errorcluster)  [unwired: 1 in]
      n125 = property class="TabCtl (strict)"(reference=w219, "Visible"=FALSE) -> (reference out=w218:refnum<vi>, error out=w220:errorcluster)  [unwired: 1 in]
      n126 = property class="Bool (strict)"(reference=w206, "Visible"=FALSE) -> (reference out=w205:refnum<vi>, error out=w207:errorcluster)  [unwired: 1 in]
      n127 = property class="DigNum (strict)"(reference=w203, "Visible"=FALSE) -> (reference out=w204:refnum<vi>, error out=w202:errorcluster)  [unwired: 1 in]
      n128 = property class="DigNum (strict)"(reference=w200, "Visible"=FALSE) -> (reference out=w199:refnum<vi>, error out=w201:errorcluster)  [unwired: 1 in]
      n129 = property class="Ring (strict)"(reference=w208, "Visible"=FALSE) -> (reference out=w213:refnum<vi>, error out=w209:errorcluster)  [unwired: 1 in]
      n130 = property class="DigNum (strict)"(reference=w211, "Visible"=FALSE) -> (reference out=w212:refnum<vi>, error out=w210:errorcluster)  [unwired: 1 in]
      n131 = property class="Ring (strict)"(reference=w214, "Visible"=FALSE) -> (reference out=w216:refnum<vi>, error out=w215:errorcluster)  [unwired: 1 in]
      n132 = property class="DigNum (strict)"(reference=w191, "Visible"=FALSE) -> (reference out=w189:refnum<vi>, error out=w190:errorcluster)  [unwired: 1 in]
      n133 = property class="Str"(reference=w171, "Visible"=FALSE) -> (reference out=w172:refnum<vi>, error out=w170:errorcluster)  [unwired: 1 in]
      n134 = property class="MCListbox (strict)"(reference=w174, "Visible"=FALSE) -> (reference out=w173:refnum<vi>, error out=w175:errorcluster)  [unwired: 1 in]
      n135 = property class="DigNum (strict)"(reference=w177, "Visible"=FALSE) -> (reference out=w178:refnum<vi>, error out=w176:errorcluster)  [unwired: 1 in]
      n136 = property class="DigNum (strict)"(reference=w169, "Visible"=FALSE) -> (reference out=w164:refnum<vi>, error out=w168:errorcluster)  [unwired: 1 in]
      n137 = property class="DigNum (strict)"(reference=w166, "Visible"=FALSE) -> (reference out=w165:refnum<vi>, error out=w167:errorcluster)  [unwired: 1 in]
      n138 = property class="Str"(reference=w163, "Visible"=FALSE) -> (reference out=w161:refnum<vi>, error out=w162:errorcluster)  [unwired: 1 in]
      n139 = property class="DigNum (strict)"(reference=w186, "Visible"=FALSE) -> (reference out=w188:refnum<vi>, error out=w187:errorcluster)  [unwired: 1 in]
      n140 = property class="Str"(reference=w150, "Visible"=FALSE) -> (reference out=w149:refnum<vi>, error out=w151:errorcluster)  [unwired: 1 in]
      n141 = property class="DigNum (strict)"(reference=w147, "Visible"=FALSE) -> (reference out=w148:refnum<vi>, error out=w146:errorcluster)  [unwired: 1 in]
      n142 = property class="Str"(reference=w144, "Visible"=FALSE) -> (reference out=w143:refnum<vi>, error out=w145:errorcluster)  [unwired: 1 in]
      n143 = property class="Str"(reference=w152, "Visible"=FALSE) -> (reference out=w157:refnum<vi>, error out=w153:errorcluster)  [unwired: 1 in]
      n144 = property class="Str"(reference=w155, "Visible"=FALSE) -> (reference out=w156:refnum<vi>, error out=w154:errorcluster)  [unwired: 1 in]
      n145 = property class="Str"(reference=w158, "Visible"=FALSE) -> (reference out=w160:refnum<vi>, error out=w159:errorcluster)  [unwired: 1 in]
      n146 = Close Reference(reference=w246, error in (no error)=w247) -> ()  [unwired: 1 out]
      n147 = Close Reference(reference=w245, error in (no error)=w244) -> ()  [unwired: 1 out]
      n148 = Close Reference(reference=w239, error in (no error)=w240) -> ()  [unwired: 1 out]
      n149 = Close Reference(reference=w236, error in (no error)=w235) -> ()  [unwired: 1 out]
      n150 = Close Reference(reference=w230, error in (no error)=w232) -> ()  [unwired: 1 out]
      n151 = Close Reference(reference=w226, error in (no error)=w228) -> ()  [unwired: 1 out]
      n152 = Close Reference(reference=w225, error in (no error)=w223) -> ()  [unwired: 1 out]
      n153 = Close Reference(reference=w218, error in (no error)=w220) -> ()  [unwired: 1 out]
      n154 = Close Reference(reference=w205, error in (no error)=w207) -> ()  [unwired: 1 out]
      n155 = Close Reference(reference=w204, error in (no error)=w202) -> ()  [unwired: 1 out]
      n156 = Close Reference(reference=w199, error in (no error)=w201) -> ()  [unwired: 1 out]
      n157 = Close Reference(reference=w213, error in (no error)=w209) -> ()  [unwired: 1 out]
      n158 = Close Reference(reference=w212, error in (no error)=w210) -> ()  [unwired: 1 out]
      n159 = Close Reference(reference=w216, error in (no error)=w215) -> ()  [unwired: 1 out]
      n160 = Close Reference(reference=w189, error in (no error)=w190) -> ()  [unwired: 1 out]
      n161 = Close Reference(reference=w172, error in (no error)=w170) -> ()  [unwired: 1 out]
      n162 = Close Reference(reference=w173, error in (no error)=w175) -> ()  [unwired: 1 out]
      n163 = Close Reference(reference=w178, error in (no error)=w176) -> ()  [unwired: 1 out]
      n164 = Close Reference(reference=w164, error in (no error)=w168) -> ()  [unwired: 1 out]
      n165 = Close Reference(reference=w165, error in (no error)=w167) -> ()  [unwired: 1 out]
      n166 = Close Reference(reference=w161, error in (no error)=w162) -> ()  [unwired: 1 out]
      n167 = Close Reference(reference=w188, error in (no error)=w187) -> ()  [unwired: 1 out]
      n168 = Close Reference(reference=w149, error in (no error)=w151) -> ()  [unwired: 1 out]
      n169 = Close Reference(reference=w148, error in (no error)=w146) -> ()  [unwired: 1 out]
      n170 = Close Reference(reference=w143, error in (no error)=w145) -> ()  [unwired: 1 out]
      n171 = Close Reference(reference=w157, error in (no error)=w153) -> ()  [unwired: 1 out]
      n172 = Close Reference(reference=w156, error in (no error)=w154) -> ()  [unwired: 1 out]
      n173 = Close Reference(reference=w160, error in (no error)=w159) -> ()  [unwired: 1 out]
    }
  }
  "error out" <- w10
  n174 = Unbundle By Name("Data Cluster") -> ("Motion Module.M3 Image"=w11:refnum<vi>)
  n175 = Unbundle By Name("Data Cluster") -> ("Main Home Screen.MainPage"=w8:refnum<vi>)
  n176 = property class="TabCtl (strict)"(reference=w11, "Value"=enum32{"Page 1", "Page 2"}."Page 1") -> (reference out=w13:refnum<vi>, error out=w12:errorcluster)  [unwired: 1 in]
  n177 = Unbundle By Name("Data Cluster") -> ("Main Home Screen.GUI"=w4:refnum<vi>)
  n178 = property class="TabCtl (strict)"(reference=w8, "Value"=T2."HOME") -> (reference out=w6:refnum<vi>, error out=w7:errorcluster)  [unwired: 1 in]
  n179 = property class="TabCtl (strict)"(reference=w4, "Value"=T3."Motion Module") -> (reference out=w2:refnum<vi>, error out=w3:errorcluster)  [unwired: 1 in]
  n180 = Close Reference(reference=w13, error in (no error)=w12) -> ()  [unwired: 1 out]
  n181 = Close Reference(reference=w6, error in (no error)=w7) -> ()  [unwired: 1 out]
  n182 = Close Reference(reference=w2, error in (no error)=w3) -> ()  [unwired: 1 out]
